vi "Get SMO Database Paths.vi"(5 "getAll Cluster":variant, 7 "Default Paths":string, 8 "error in (no error)":errorcluster, 11 "Instrument in":refnum<class "Instrument.lvclass">) -> (0 "error out":errorcluster, 2 "Paths":string, 3 "Instrument out":refnum<class "Instrument.lvclass">)   [LabVIEW 2019, in "Instrument.lvclass"]
doc: "Override this VI to return a list of paths for logging data"
uses:
  Instrument.lvclass
  Instrument.lvclass/Instrument.ctl
  <userlib>/LevyLab/LV-Data/LV-Data.PG/LV-Data.PGSQL.lvclass
  <vilib>/Utility/Data Type/NI_Data Type.lvlib
  <userlib>/LevyLab/LV-Data/LV-Data.PG/API/Write Variable (one-row).vi
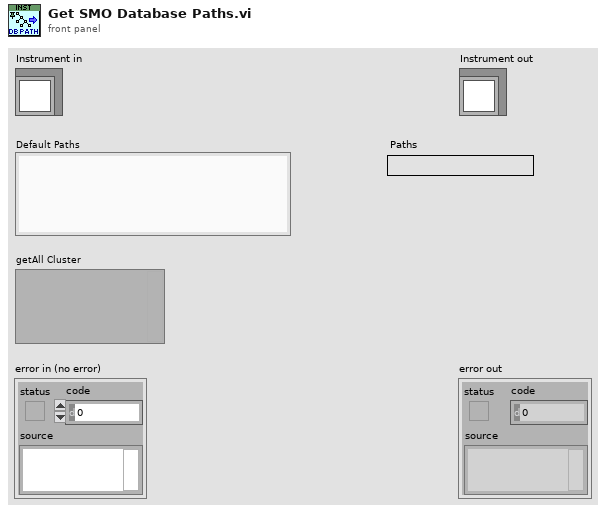
[diagram p1: front panel]
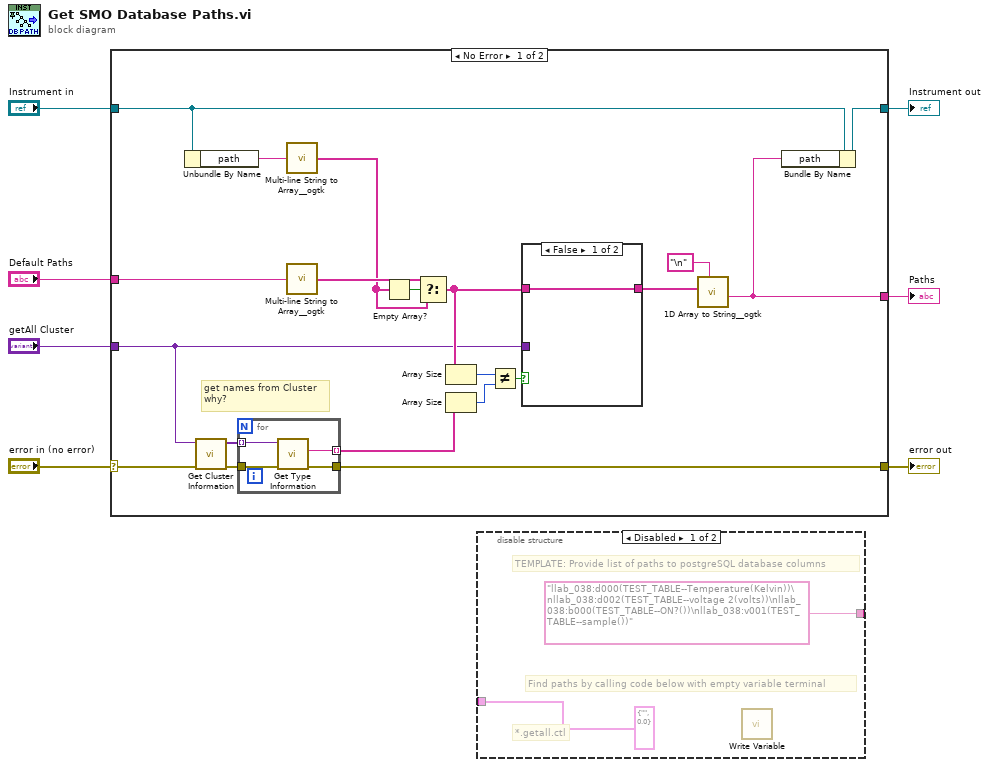
[diagram p0: block diagram]
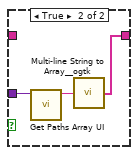
[diagram p2: hidden frame]
diagram:
  n1 = case shown="No Error" "error in (no error)" {
    selector: "error in (no error)" -> [w12 w37]
    tunnel: [w15 w37] -> w6
    tunnel: [w26 w36] -> w4
    tunnel: "Instrument in" -> [w27 w36]
    tunnel: "Default Paths" -> [w24 _]
    tunnel: [w8 _] -> w2
    tunnel: "getAll Cluster" -> [w14 _]
    frame No Error {
      # "get names from Cluster\nwhy?"
      n2 = Unbundle By Name(w27) -> ("path"=w11:string)
      n3 = call <vilib>:"Get Cluster Information.vi"("error in (no error)"=w12, "variant"=w14) -> ("error out"=w16:errorcluster, "cluster elements"=w17:variant[])  [unwired: 8 in]
      n4 = for {
        tunnel: w17 -> [w31] mode=indexing
        tunnel: w16 -> [w30]
        tunnel: [w29] -> w15
        tunnel: [w28] -> w13 mode=indexing
        n5 = call <vilib>:"Get Type Information.vi"("error in (no error)"=w30, "variant"=w31) -> ("error out"=w29:errorcluster, "name"=w28:string)  [unwired: 5 in, 3 out]
      }
      n6 = call <userlib>:"Multi-line String to Array__ogtk.vi"("string"=w11) -> ("lines"=w10:string[])
      n7 = call <userlib>:"Multi-line String to Array__ogtk.vi"("string"=w24) -> ("lines"=w22:string[])
      n8 = Empty Array?(array=w10) -> (empty?=w25:bool)
      n9 = Select(t=w22, s=w25, f=w10) -> (s? t:f=w19:string[])
      n10 = Array Size(array=w19) -> (size(s)=w18:i32)
      n11 = Array Size(array=w13) -> (size(s)=w21:i32)
      n12 = Not Equal?(x=w18, y=w21) -> (x != y?=w20:bool)
      n13 = case shown="False" w20 {
        tunnel: w14 -> [_ w35]
        tunnel: [w32 w33] -> w9
        tunnel: w19 -> [w32 _]
        frame False {
        }
        frame True {
          n14 = call <userlib>:"Get Paths Array UI.vi"("Data"=w35) -> ("selected_paths"=w34:string)  [unwired: 9 in, 1 out]
          n15 = call <userlib>:"Multi-line String to Array__ogtk.vi"("string"=w34) -> ("lines"=w33:string[])
        }
      }
      n16 = call <userlib>:"1D Array to String__ogtk.vi"("delimiter (Tab)"="\n", "Array of Strings"=w9) -> ("delimited string"=w8:string)  [unwired: 9 in]
      n17 = Bundle By Name(cluster=w27, "path"=w8) -> (w26:refnum<class "Instrument.lvclass">)
    }
    frame Error {
    }
  }
  "error out" <- w6
  "Instrument out" <- w4
  "Paths" <- w2
  n18 = disable-structure shown="Disabled" {
    disable-tunnel: ["llab_038:d000(TEST_TABLE--Temperature(Kelvin))\nllab_038:d002(TEST_TABLE--voltage 2(volts))\nllab_038:b000(TEST_TABLE--ON?())\nllab_038:v001(TEST_TABLE--sample())" ("Paths") _] -> _
    disable-tunnel: [cluster{string, dbl} {"", 0.0} _] -> _
    frame Disabled {
      # "Find paths by calling code below with empty variable terminal"
      # "*.getall.ctl"
      # "TEMPLATE: Provide list of paths to postgreSQL database columns"
      n19 = call-poly <userlib>:"Write Variable.vi"() -> ()  [unwired: 8 in, 4 out]
    }
    frame Enabled {
    }
  }
